vi "N147x_charge_transport.vi"() -> ()   [LabVIEW 2019]
uses:
  <vilib>/Analysis/baseanly.llb/Mean (DBL).vi
  <vilib>/Utility/file.llb/Write To Spreadsheet File (DBL).vi
  N471A.lvlib
  Users/pcmmegas02/Downloads/CAEN_PSM-InstrumentDriver-1.0.2/CAEN PSM/CAEN PSM.lvlib
  <vilib>/Analysis/NI_AALBase.lvlib
  <vilib>/gmath/NI_Gmath.lvlib
panel:
  out "seconds since 1Jan1904":timestamp
  in  "one time average":bool
  out "IMon Graph":cluster{"Y":dbl[], "Y":dbl[]}[](graph)
  out "VMon Graph":cluster{"Y":dbl[], "Y":dbl[]}[](graph)
  out "Mean-St.dev. 1":dbl[](array[numeric]) format="%#.2g"
  out "Mean-St.dev. 2":dbl[](array[numeric]) format="%#.2g"
  out "Mean-St.dev. 3":dbl[](array[numeric]) format="%#.2g"
  out "Mean-St.dev. 4":dbl[](array[numeric]) format="%#.2g"
  out "IMON RT 1":dbl[](array[numeric])
  out "IMON RT 2":dbl[](array[numeric])
  out "IMON RT 3":dbl[](array[numeric])
  out "IMON RT 4":dbl[](array[numeric])
  out "VMON RT 1":dbl[](array[numeric])
  out "VMON RT 2":dbl[](array[numeric])
  out "VMON RT 3":dbl[](array[numeric])
  out "VMON RT 4":dbl[](array[numeric])
  in  "Average length":i32=50
  out "Board Handle":T1
  in  "Save":bool
  out "Time Array":dbl[](array[numeric])=[0.09375, 0.46875, 0.84375, 1.78125, 2.15625, 2.53125, 2.921875, 3.28125, 6.09375, 6.46875, 6.859375, 7.234375, 7.609375, 7.984375, 8.359375, 8.734375, 9.109375, 9.484375, 9.859375, 10.234375, 10.625, 10.984375, 11.375, 11.75, 12.125, 12.5, 12.875, 13.25, 13.625, 14.0, 14.390625, 14.765625, 15.140625, 15.515625, 15.890625, 16.265625, 16.640625, 17.015625, 17.390625, 17.765625, 18.140625, 18.515625, 18.90625, 19.28125, 19.65625, 20.03125, 20.40625, 20.78125, 21.15625, 21.53125, 21.90625, 22.28125, 22.65625, 23.046875, 23.421875, 23.796875, 24.171875, 24.546875, 24.921875, 25.296875, 25.671875, 26.0625, 26.4375, 26.8125, 27.1875, 27.5625, 27.9375, 28.3125, 28.6875, 29.0625, 29.4375, 29.8125, 30.203125, 30.578125, 30.953125, 31.328125, 31.703125, 32.078125, 32.453125, 32.828125, 33.203125, 33.578125, 33.96875, 34.34375, 34.71875, 35.09375, 37.96875, 38.34375, 38.71875, 39.09375, 39.46875, 39.84375, 40.21875, 40.59375, 40.96875, 41.34375, 41.71875, 42.09375, 42.484375, 42.859375, 43.234375, 43.609375, 43.984375, 44.359375, 44.734375, 45.109375, 45.484375, 45.859375, 46.25, 46.625, 47.0, 47.375, 47.75, 48.125, 48.5, 48.875, 49.265625, 49.640625, 50.015625, 50.390625, 50.765625, 51.140625, 51.515625, 51.890625, 52.265625, 52.640625, 53.015625, 53.390625, 53.765625, 54.15625, 54.53125, 54.90625, 55.28125, 55.65625, 56.03125, 56.40625, 56.78125, 57.15625, 57.53125, 57.921875, 58.296875, 58.671875, 59.046875, 59.421875, 59.796875, 60.171875, 60.546875, 60.9375, 61.296875, 61.6875, 62.0625, 62.4375, 62.8125, 63.1875, 63.5625, 63.9375, 64.3125, 64.6875, 65.0625, 65.4375, 65.828125, 66.203125, 66.578125, 66.953125, 67.328125, 67.703125, 68.078125, 68.453125, 68.84375, 69.21875, 69.59375, 69.96875, 70.34375, 70.71875, 71.09375, 71.46875, 71.84375, 72.21875, 72.59375, 72.984375, 73.359375, 73.734375, 74.109375, 74.484375, 74.859375, 75.234375, 75.609375, 75.984375, 76.359375, 76.734375, 77.109375, 77.5, 77.875, 78.25, 78.625, 79.0, 79.375, 79.75, 80.125, 80.515625, 80.890625, 81.265625]
  out "IMON Array":dbl[][](array[numeric])
  out "VMON Array":dbl[][](array[numeric])
  in  "stop":bool
  in  "Module Address":u16(ring) items=["0", "1", "2", "3", "4", "5", "6", "7", "8", "9", "10", "11", "12", "13", "14", "15", "16", "17", "18", "19", "20", "21", "22", "23", "24", "25", "26", "27", "28", "29", "30", "31"]
  in  "VISA resource name in":refnum<visa-resource-name>="COM13"
  out "error out":errorcluster
  in  "N147x":T2(tab)
  in  "Read Status and Configuration":bool
  out "Name":string
  out "Number Of Channels":string
  out "Firmware Release":string
  out "Serial Number":string
  out "Channel Status Array":T3(array[cluster])
  out "PWDW":string[](array[string])
  out "Polarity":string[](array[string])
  out "MAXV":i32[](array[numeric])
  out "RDW":i32[](array[numeric])
  out "RUP":i32[](array[numeric])
  out "IMON":dbl[](array[numeric]) format="%.1f"
  out "ISET":dbl[](array[numeric]) format="%.1f"
  out "VMON":dbl[](array[numeric]) format="%.1f"
  out "VSET":dbl[](array[numeric]) format="%.1f"
  out "Number of Channel Detected":u8=4
  out "Monitoring Error":bool
  in  "IMon range":string(combo)="KILL"
  in  "Power down":string(combo)="KILL"
  in  "ALL OFF":bool
  in  "ALL ON":bool
  in  "Channels ON/OFF":bool[](array[boolean])=[TRUE, TRUE, TRUE, TRUE]
  in  "IM RANGE":bool
  in  "PDWN":bool
  in  "TRIP":bool
  in  "RDW":bool
  in  "RUP":bool
  in  "MAXV":bool
  in  "ISET[uA]":bool
  in  "VSET":bool
  in  "Channels Selection":bool[](array[boolean])=[FALSE, FALSE, FALSE, FALSE]
  in  "Upload Values":bool
  in  "Set V":dbl format="%06.1f"
  in  "Set I":dbl=2.0 format="%07.3f"
  in  "Set Max V":dbl=1000.0 format="%04.0f"
  in  "Set Ramp Up":dbl=10.0 format="%03.0f"
  in  "Set Ramp Down":dbl=50.0 format="%03.0f"
  in  "Set Trip":dbl=1000.0 format="%06.1f"
  in  "Update On/OFF":bool
  out "Error  on \nChannels \nON/OFF":bool
  out "IMon  RT Err":bool
  out "VMon  RT Err":bool
  in  "stop HV scan":bool
  in  "Waiting [s]":u32=7
  in  "Step [V]":dbl[](array[numeric])=[50.0, 50.0] format="%06.1f"
  in  "Vstop":dbl[](array[numeric])=[1600.0, 1600.0, 10.0, 10.0] format="%06.1f"
  in  "Channels Selection 2":bool[](array[boolean])=[FALSE, FALSE, FALSE, FALSE]
  in  "Start HV scan":bool
  in  "Vstart":dbl[](array[numeric])=[0.0, 0.0, 10.0, 10.0] format="%06.1f"
  in  "pts/step":i32=5
  out "logged pts/step":i32
  out "Scatter Plot":cluster{dbl[], dbl[]}[](graph)=[{[199.2, 172.7, 149.1, 124.2, 99.2, 74.2, 49.19999999999999, 24.30000000000001, -0.5999999999999943, -25.5, -50.5, -75.39999999999998, -100.39999999999998, -125.5, -150.3, -175.2, -200.2, -225.2, -250.10000000000002, -275.1, -300.2, -325.0, -350.0, -375.0, -399.9, -424.70000000000005, -449.70000000000005, -474.6, -499.70000000000005, -524.8000000000001, -549.8000000000001, -574.6, -599.4, -599.6, -599.6, -599.6, -599.6, -599.6, -599.6], [0.0, 0.0, 0.0, 0.0, 0.0, 0.0, 0.0, 0.05, 0.05, 0.05, 0.05, 0.15, 0.1, 0.15, 0.15, 0.15, 0.15, 0.2, 0.2, 0.25, 0.25, 0.3, 0.35, 0.4, 0.4, 0.4, 0.45, 0.5, 0.45, 0.5, 0.55, 0.6, 0.6, 0.6, 0.65, 0.6, 0.6, 0.6, 0.6]}, {[199.2, 172.7, 149.1, 124.2, 99.2, 74.2, 49.19999999999999, 24.30000000000001, -0.5999999999999943, -25.5, -50.5, -75.39999999999998, -100.39999999999998, -125.5, -150.3, -175.2, -200.2, -225.2, -250.10000000000002, -275.1, -300.2, -325.0, -350.0, -375.0, -399.9, -424.70000000000005, -449.70000000000005, -474.6, -499.70000000000005, -524.8000000000001, -549.8000000000001, -574.6, -599.4, -599.6, -599.6, -599.6, -599.6, -599.6, -599.6], [0.1, 0.25, 0.15, 0.15, 0.15, 0.2, 0.2, 0.25, 0.25, 0.25, 0.25, 0.3, 0.35, 0.4, 0.4, 0.45, 0.5, 0.5, 0.6, 0.65, 0.75, 0.9, 1.0, 1.15, 1.3, 1.5, 1.8, 2.1, 2.4499999999999997, 2.9499999999999997, 3.4499999999999997, 4.2, 5.05, 5.05, 5.05, 5.05, 5.1000000000000005, 5.15, 5.1000000000000005]}, {[199.2, 172.7, 149.1, 124.2, 99.2, 74.2, 49.19999999999999, 24.30000000000001, -0.5999999999999943, -25.5, -50.5, -75.39999999999998, -100.39999999999998, -125.5, -150.3, -175.2, -200.2, -225.2, -250.10000000000002, -275.1, -300.2, -325.0, -350.0, -375.0, -399.9, -424.70000000000005, -449.70000000000005, -474.6, -499.70000000000005, -524.8000000000001, -549.8000000000001, -574.6, -599.4, -599.6, -599.6, -599.6, -599.6, -599.6, -599.6], [0.0, 0.6, 0.05, 0.05, 0.05, 0.05, 0.05, 0.05, 0.05, 0.1, 0.1, 0.1, 0.15, 0.1, 0.15, 0.15, 0.15, 0.15, 0.15, 0.2, 0.2, 0.25, 0.25, 0.3, 0.35, 0.45, 0.5, 0.6, 0.7, 0.8, 1.0, 1.2, 1.55, 1.5, 1.5, 1.45, 1.5, 1.45, 1.45]}, {[199.2, 172.7, 149.1, 124.2, 99.2, 74.2, 49.19999999999999, 24.30000000000001, -0.5999999999999943, -25.5, -50.5, -75.39999999999998, -100.39999999999998, -125.5, -150.3, -175.2, -200.2, -225.2, -250.10000000000002, -275.1, -300.2, -325.0, -350.0, -375.0, -399.9, -424.70000000000005, -449.70000000000005, -474.6, -499.70000000000005, -524.8000000000001, -549.8000000000001, -574.6, -599.4, -599.6, -599.6, -599.6, -599.6, -599.6, -599.6], [0.0, 0.05, 0.1, 0.1, 0.25, 0.25, 0.25, 0.25, 0.25, 0.35, 0.35, 0.45, 0.45, 0.45, 0.5, 0.55, 0.65, 0.7, 0.8, 0.9, 0.95, 1.05, 1.2, 1.35, 1.45, 1.7, 1.9, 2.15, 2.4499999999999997, 2.8, 3.2, 3.75, 4.35, 4.3, 4.3, 4.25, 4.3, 4.3, 4.3]}]
  in  "Average values":bool
  # "Channel 1               Channel 2              Channel 3               Channel 4"
  # "VMON RT [V]"
  # "IMON RT (nA)"
  # "Mean value (nA)"
  # "St. dev."
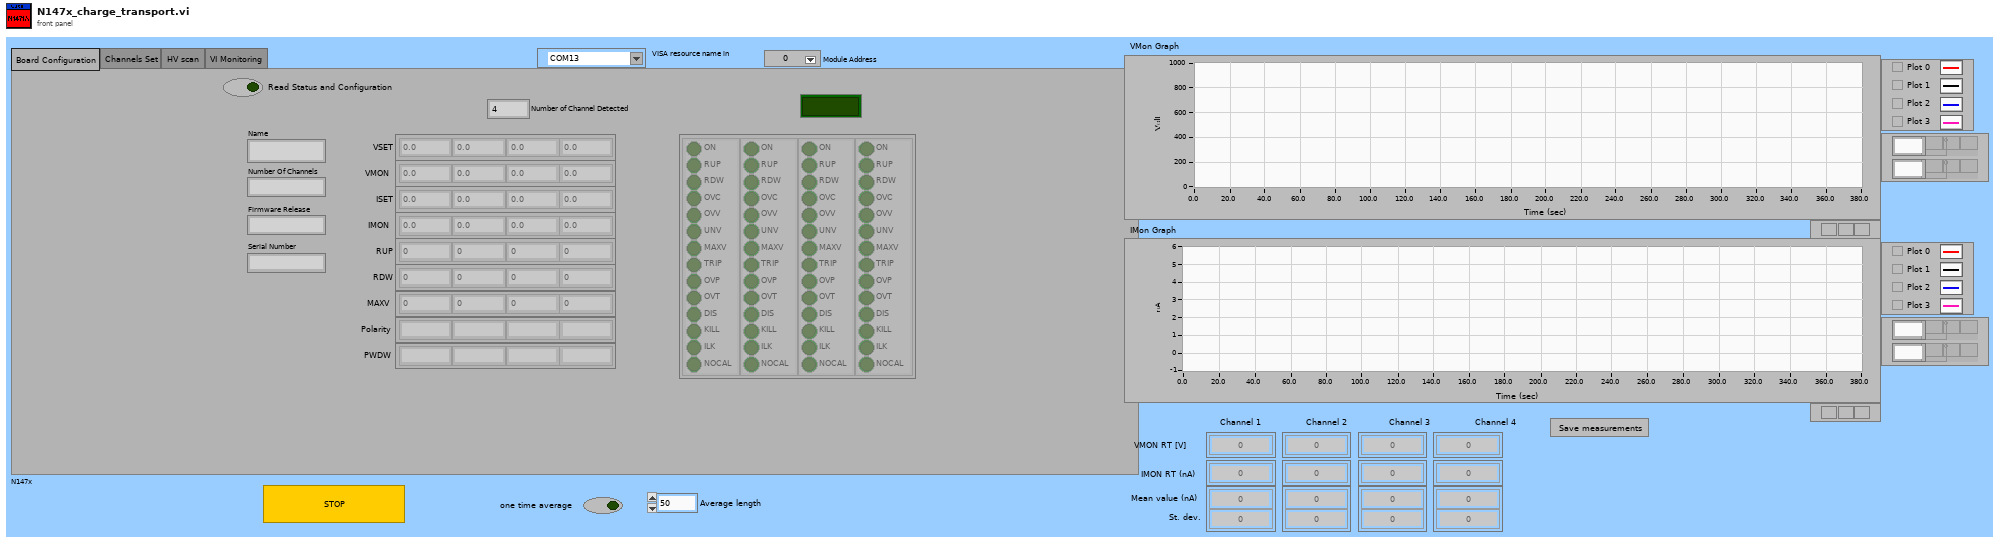
[diagram p1: front panel]
types:
  T1 = cluster{"VISA resource name in":refnum<visa-resource-name>, "Module Address":u16, "Number of Channel Detected":u8}
  T2 = enum32{"Board Configuration", "Channels Set", "HV scan", "VI Monitoring"}
  T3 = cluster{"ON":bool, "RUP":bool, "RDW":bool, "OVC":bool, "OVV":bool, "UNV":bool, "MAXV":bool, "TRIP":bool, "OVP":bool, "OVT":bool, "DIS":bool, "KILL":bool, "ILK":bool, "NOCAL":bool}[]
  T4 = cluster{"Name":string, "Num. Channels":string, "Firmware Release":string, "Serial Num.":string}
  T5 = typedef "CAEN PSM.lvlib/BoardHandle.ctl" = cluster{"VISA resource name":refnum<visa-resource-name>, "Board address":u8, "NChannels":u8}
  T6 = cluster{"ON":bool, "RUP":bool, "RDW":bool, "OVC":bool, "OVV":bool, "UNV":bool, "MAXV":bool, "TRIP":bool, "OVP":bool, "OVT":bool, "DIS":bool, "KILL":bool, "ILK":bool, "NOCAL":bool}
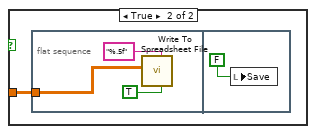
[diagram p3: hidden frame]
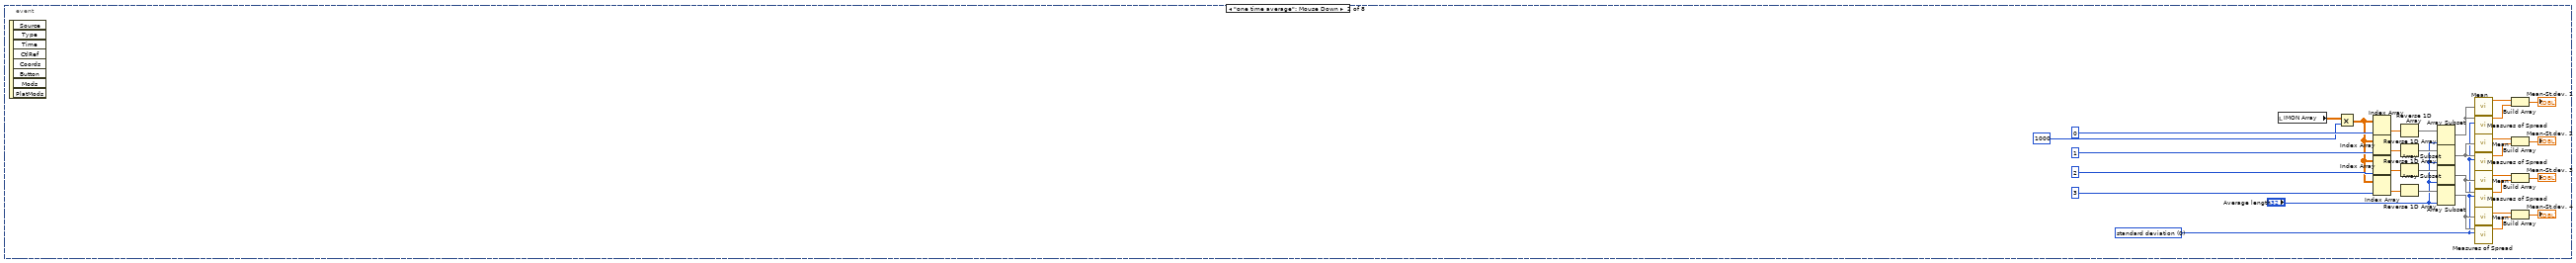
[diagram p4: hidden frame]
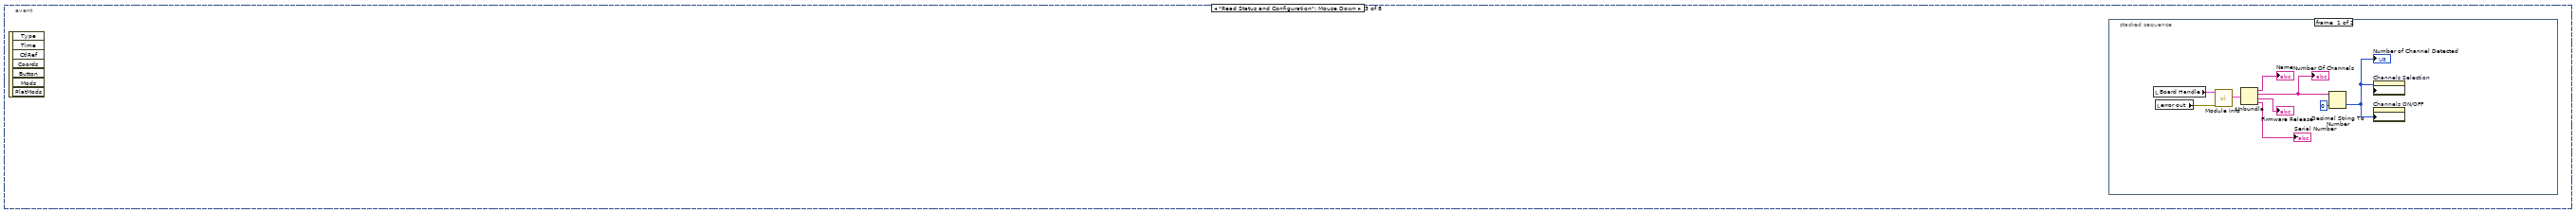
[diagram p5: hidden frame]
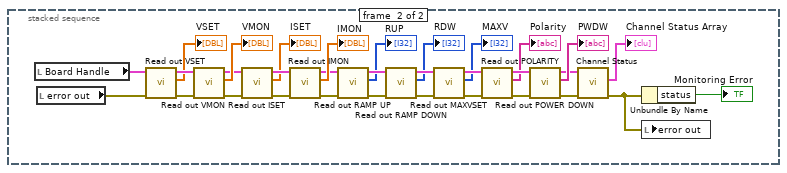
[diagram p6: hidden frame]
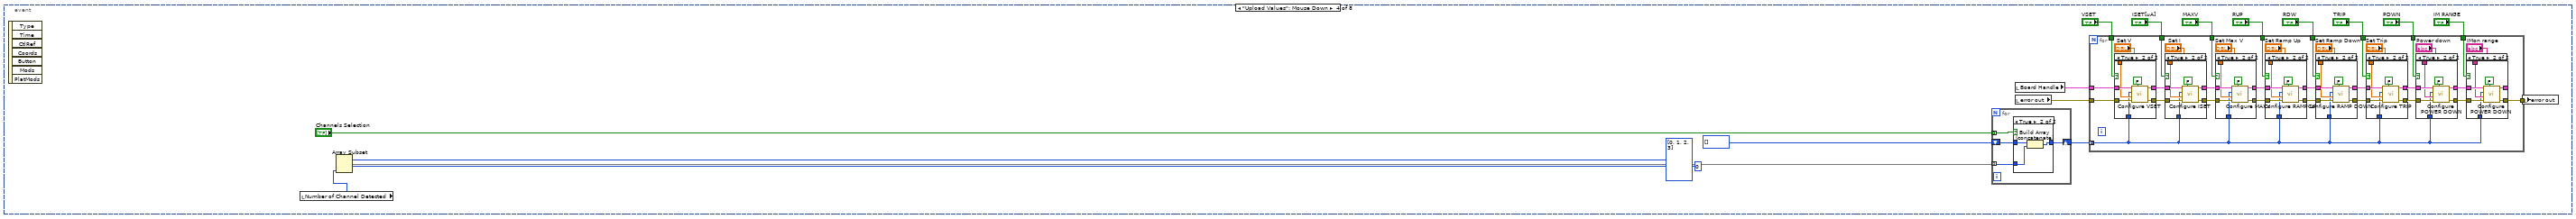
[diagram p7: hidden frame]
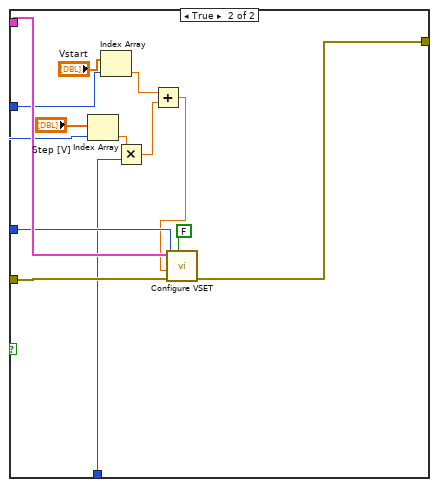
[diagram p18: hidden frame]
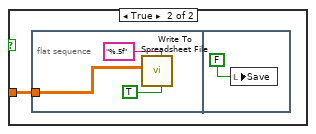
[diagram p19: hidden frame]
diagram:
  n1 = call "Initialize.vi"("VISA resource name"="VISA resource name in") -> ("error out"=w13:errorcluster, "VISA resource name out"=w9:refnum<visa-resource-name>)  [unwired: 9 in]
  n2 = local read "Number of Channel Detected"() -> (w6:u8)
  n3 = local read "VISA resource name in"() -> (w7:refnum<visa-resource-name>)
  n4 = local read "Module Address"() -> (w5:u16)
  n5 = call "OpenBoard.vi"("error in (no error)"=w13, "Board Address"=w5, "VISA resource name"=w9) -> ("error out"=w10:errorcluster)  [unwired: 7 in, 1 out]
  n6 = flat-sequence {
    tunnel: w10 -> [w17]
    tunnel: [w16] -> w11
    tunnel: [w22] -> w12
    tunnel: w11 -> [w22]
    tunnel: [w20] -> w1
    frame #0 {
      n7 = call "Display Message to User"("error in (no error)"=w17) -> ("error out"=w16:errorcluster)  [unwired: 9 in, 1 out]
    }
    frame #1 {
      w19 = dbl[][] [] ("VMON Array")
      n8 = local write "VMON Array"(w19) -> ()
      n9 = local write "IMON Array"(w19) -> ()
      n10 = local write "Time Array"(dbl[] [] ("Time Array")) -> ()
      n11 = local write "N147x"(enum32{"Board Configuration", "Channels Set"}."Board Configuration" ("N1471A 2")) -> ()
      n12 = Get Date/Time In Seconds() -> (seconds since 1Jan1904=w20:timestamp)
    }
  }
  n13 = Bundle("VISA resource name in"=w7, "Module Address"=w5, "Number of Channel Detected"=w6) -> (w8:T1)  [unwired: 1 in]
  "Board Handle" <- w8
  n14 = local write "Board Handle"(w8) -> ()
  n15 = while {
    shift-right: [w23] -> w4
    shift-left: w12 -> [w28]
    tunnel: [FALSE ("stop")] -> w15
    stop <- w26 stop-if-true
    n16 = flat-sequence {
      tunnel: w28 -> [w30]
      tunnel: [w30] -> w29
      frame #0 {
        n17 = local write "error out"(w30) -> ()
      }
    }
    n18 = case shown="No Error" w29 {
      selector: w29 -> [_ w821]
      tunnel: [w31 w821] -> w23
      frame No Error {
        n19 = event shown="[4] \"Start HV scan\": Mouse Down" {
          selector: _ -> [_ _ _ _ _ _ _ _]
          dyn-events: _ -> [_ _ _ _ _ _ _ _]
          timeout: u32 1 ("Time") -> [_ _ _ _ _ _ _ _]
          tunnel: [w100 _ _ _ _ _ _ _] -> w31
          event Timeout {
            w91 = cluster{dbl[], dbl[]}[] []
            w99 = FALSE ("Open/Close [T]")
            n20 = event-data() -> ()  [unwired: 1 in, 2 out]
            n21 = local read "Number of Channel Detected"() -> (w88:u8)
            n22 = local read "seconds since 1Jan1904"() -> (w33:timestamp)
            n23 = Get Date/Time In Seconds() -> (seconds since 1Jan1904=w95:timestamp)
            n24 = local read "VISA resource name in"() -> (w103:refnum<visa-resource-name>)
            n25 = local read "Module Address"() -> (w98:u16)
            n26 = local read "VMON Array"() -> (w87:dbl[][])
            n27 = local read "IMON Array"() -> (w92:dbl[][])
            n28 = Subtract(x=w95, y=w33) -> (x-y=w89:dbl)
            n29 = local read "Time Array"() -> (w90:dbl[])
            n30 = Wait Until Next ms Multiple(millisecond multiple=u32 1000 ("milliseconds to wait")) -> ()  [unwired: 1 out]
            n31 = Build Array (concatenate)(w90, w89) -> (w75:dbl[])
            n32 = local write "Time Array"(w75) -> ()
            n33 = local read "error out"() -> (w63:errorcluster)
            n34 = call "N1471A-MonitorVMON.vi"("VISA resource name in"=w103, "Module Address"=w98, "Channel"=w88, "error in (no error)"=w63, "Open/Close [T]"=w99) -> ("VISA resource name out"=w102:refnum<visa-resource-name>, "Error"=→"VMon  RT Err":bool, "Values"=w94:string[], "error out"=w101:errorcluster)  [unwired: 9 in, 2 out]
            n35 = call "N1471A-MonitorIMON.vi"("VISA resource name in"=w102, "Module Address"=w98, "Channel"=w88, "error in (no error)"=w101, "Open/Close [T]"=w99) -> ("Error"=→"IMon  RT Err":bool, "Values"=w93:string[], "error out"=w100:errorcluster)  [unwired: 9 in, 3 out]
            n36 = for {
              N: w88 -> [_]
              tunnel: w94 -> [w130] mode=indexing
              tunnel: w93 -> [w127] mode=indexing
              tunnel: [w129] -> w34 mode=indexing
              tunnel: [w128] -> w53 mode=indexing
              tunnel: w92 -> [w122]
              tunnel: w87 -> [w124]
              i -> [w121]
              n37 = Index Array(array=w124, index (col)=w121) -> (element=w123:dbl[])  [unwired: 1 in]
              n38 = Index Array(array=w122, index (col)=w121) -> (element=w120:dbl[])  [unwired: 1 in]
              n39 = Fract/Exp String To Number(string=w130) -> (number=w126:dbl)  [unwired: 3 in, 1 out]
              n40 = Fract/Exp String To Number(string=w127) -> (number=w125:dbl)  [unwired: 3 in, 1 out]
              n41 = Build Array (concatenate)(w123, w126) -> (w129:dbl[])
              n42 = Build Array (concatenate)(w120, w125) -> (w128:dbl[])
            }
            n43 = Multiply(x=w53, y=1000) -> (x*y=w48:dbl[][])
            n44 = Index Array(array=w34, index (row) #1=0 ("index (row)"), index (row) #2=1 ("index (row)"), index (row) #3=2 ("index (row)"), index (row) #4=3 ("index (row)")) -> (element #1=w74:dbl[], element #2=w72:dbl[], element #3=w70:dbl[], element #4=w68:dbl[])  [unwired: 4 in]
            n45 = Index Array(array=w53, index (row) #1=0 ("index (row)"), index (row) #2=1 ("index (row)"), index (row) #3=2 ("index (row)"), index (row) #4=3 ("index (row)")) -> (element #1=w73:dbl[], element #2=w71:dbl[], element #3=w69:dbl[], element #4=w67:dbl[])  [unwired: 4 in]
            n46 = Transpose 2D Array(2D array=w34) -> (transposed array=w86:dbl[][])
            n47 = Transpose 2D Array(2D array=w53) -> (transposed array=w62:dbl[][])
            n48 = Index Array(array=w48, index (row) #1=0 ("index (row)"), index (row) #2=1 ("index (row)"), index (row) #3=2 ("index (row)"), index (row) #4=3 ("index (row)")) -> (element #1=w57:dbl[], element #2=w56:dbl[], element #3=w55:dbl[], element #4=w54:dbl[])  [unwired: 4 in]
            n49 = Build Array(w75, w74, w73, w72, w71, w70, w69, w68, w67) -> (w66:dbl[][])
            n50 = local write "VMON Array"(w86) -> ()
            n51 = local write "IMON Array"(w62) -> ()
            n52 = Reverse 1D Array(array=w57) -> (reversed array=→"IMON RT 1":dbl[])
            n53 = Reverse 1D Array(array=w56) -> (reversed array=→"IMON RT 2":dbl[])
            n54 = Reverse 1D Array(array=w55) -> (reversed array=→"IMON RT 3":dbl[])
            n55 = Reverse 1D Array(array=w54) -> (reversed array=→"IMON RT 4":dbl[])
            n56 = case shown="False" "Save" {
              tunnel: w66 -> [_ w104]
              frame False {
              }
              frame True {
                n57 = flat-sequence {
                  tunnel: w104 -> [w106]
                  frame #0 {
                    n58 = call-poly <vilib>:"Write To Spreadsheet File.vi"("transpose? (no:F)"=TRUE, "format (%.3f)"="%.5f", "2D data"=w106) -> ()  [unwired: 5 in, 1 out]
                  }
                  frame #1 {
                    n59 = local write "Save"(FALSE ("Save")) -> ()
                  }
                }
              }
            }
            n60 = for {
              tunnel: w34 -> [w115] mode=indexing
              shift-right: [w119] -> w64
              shift-left: w91 -> [w118]
              shift-right: [w117] -> w85
              shift-left: w91 -> [w116]
              tunnel: w53 -> [w114] mode=indexing
              tunnel: w75 -> [w113]
              n61 = Multiply(x=w114, y=1000) -> (x*y=w110:dbl[])
              n62 = Bundle(w113, w115) -> (w112:cluster{dbl[], dbl[]})  [unwired: 1 in]
              n63 = Bundle(w113, w110) -> (w111:cluster{dbl[], dbl[]})  [unwired: 1 in]
              n64 = Build Array (concatenate)(w118, w112) -> (w119:cluster{dbl[], dbl[]}[])
              n65 = Build Array (concatenate)(w116, w111) -> (w117:cluster{dbl[], dbl[]}[])
            }
            "IMon Graph" <- w85
            "VMon Graph" <- w64
            n66 = Index Array(array=w34, index (row) #1=0 ("index (row)"), index (row) #2=1 ("index (row)"), index (row) #3=2 ("index (row)"), index (row) #4=3 ("index (row)")) -> (element #1=w42:dbl[], element #2=w41:dbl[], element #3=w40:dbl[], element #4=w39:dbl[])  [unwired: 4 in]
            n67 = Reverse 1D Array(array=w42) -> (reversed array=→"VMON RT 1":dbl[])
            n68 = Reverse 1D Array(array=w41) -> (reversed array=→"VMON RT 2":dbl[])
            n69 = Reverse 1D Array(array=w40) -> (reversed array=→"VMON RT 3":dbl[])
            n70 = Reverse 1D Array(array=w39) -> (reversed array=→"VMON RT 4":dbl[])
          }
          event "one time average": Mouse Down {
            w133 = 0 items=["standard deviation", "range", "mean absolute deviation", "interquartile range"] ("type")
            n71 = event-data() -> ()  [unwired: 1 in, 8 out]
            n72 = local read "IMON Array"() -> (w132:dbl[][])
            n73 = Multiply(x=w132, y=1000) -> (x*y=w134:dbl[][])
            n74 = Index Array(array=w134, index (col)=0 ("disabled index (col)")) -> (element=w159:dbl[])  [unwired: 1 in]
            n75 = Index Array(array=w134, index (col)=1 ("disabled index (col)")) -> (element=w158:dbl[])  [unwired: 1 in]
            n76 = Index Array(array=w134, index (col)=2 ("disabled index (col)")) -> (element=w157:dbl[])  [unwired: 1 in]
            n77 = Index Array(array=w134, index (col)=3 ("disabled index (col)")) -> (element=w156:dbl[])  [unwired: 1 in]
            n78 = Reverse 1D Array(array=w159) -> (reversed array=w154:dbl[])
            n79 = Reverse 1D Array(array=w158) -> (reversed array=w153:dbl[])
            n80 = Reverse 1D Array(array=w157) -> (reversed array=w152:dbl[])
            n81 = Reverse 1D Array(array=w156) -> (reversed array=w151:dbl[])
            n82 = Array Subset(array=w154, length="Average length") -> (w143:dbl[])  [unwired: 1 in]
            n83 = Array Subset(array=w153, length="Average length") -> (w146:dbl[])  [unwired: 1 in]
            n84 = Array Subset(array=w152, length="Average length") -> (w145:dbl[])  [unwired: 1 in]
            n85 = Array Subset(array=w151, length="Average length") -> (w144:dbl[])  [unwired: 1 in]
            n86 = call-poly <vilib>:"Mean.vi"("X"=w143) -> ("mean"=w142:dbl)  [unwired: 1 out]
            n87 = call <vilib>:"Measures of Spread.vi"("type"=w133, "x array"=w143) -> ("spread value"=w141:dbl)  [unwired: 8 in, 1 out]
            n88 = call-poly <vilib>:"Mean.vi"("X"=w146) -> ("mean"=w140:dbl)  [unwired: 1 out]
            n89 = call <vilib>:"Measures of Spread.vi"("type"=w133, "x array"=w146) -> ("spread value"=w139:dbl)  [unwired: 8 in, 1 out]
            n90 = call-poly <vilib>:"Mean.vi"("X"=w145) -> ("mean"=w138:dbl)  [unwired: 1 out]
            n91 = call <vilib>:"Measures of Spread.vi"("type"=w133, "x array"=w145) -> ("spread value"=w137:dbl)  [unwired: 8 in, 1 out]
            n92 = call-poly <vilib>:"Mean.vi"("X"=w144) -> ("mean"=w136:dbl)  [unwired: 1 out]
            n93 = call <vilib>:"Measures of Spread.vi"("type"=w133, "x array"=w144) -> ("spread value"=w135:dbl)  [unwired: 8 in, 1 out]
            n94 = Build Array(w142, w141) -> (→"Mean-St.dev. 1":dbl[])
            n95 = Build Array(w140, w139) -> (→"Mean-St.dev. 2":dbl[])
            n96 = Build Array(w138, w137) -> (→"Mean-St.dev. 3":dbl[])
            n97 = Build Array(w136, w135) -> (→"Mean-St.dev. 4":dbl[])
          }
          event "Read Status and Configuration": Mouse Down {
            n98 = event-data() -> ()  [unwired: 1 in, 7 out]
            n99 = stacked-sequence {
              frame #0 {
                n100 = local read "Board Handle"() -> (w164:T1)
                n101 = local read "error out"() -> (w165:errorcluster)
                n102 = call "Module Info.vi"("error in (no error)"=w165, "BoardHandle"=w164) -> ("Module Info"=w170:T4)  [unwired: 7 in, 2 out]
                n103 = Unbundle(w170) -> ("Name"=→"Name":string, "Num. Channels"=w168:string, "Firmware Release"=→"Firmware Release":string, "Serial Num."=→"Serial Number":string)
                "Number Of Channels" <- w168
                n104 = Decimal String To Number(string=w168, default (0L)=u8 0 ("default (0 I32)")) -> (number=w171:u8)  [unwired: 1 in, 1 out]
                "Number of Channel Detected" <- w171
                n105 = property on="Channels Selection" class="Arr (strict)"("Number of Columns"=w171) -> ()  [unwired: 2 in, 2 out]
                n106 = property on="Channels ON/OFF" class="Arr (strict)"("Number of Columns"=w171) -> ()  [unwired: 2 in, 2 out]
              }
              frame #1 {
                n107 = local read "Board Handle"() -> (w173:T1)
                n108 = local read "error out"() -> (w194:errorcluster)
                n109 = call "Read out VSET.vi"("error in (no error)"=w194, "BoardHandle"=w173) -> ("error out"=w203:errorcluster, "Vset values (V)"=→"VSET":dbl[], "BoardHandle out"=w204:T5)  [unwired: 6 in, 1 out]
                n110 = call "Read out VMON.vi"("error in (no error)"=w203, "BoardHandle"=w204) -> ("error out"=w199:errorcluster, "VMon values (V)"=→"VMON":dbl[], "BoardHandle out"=w200:T5)  [unwired: 7 in]
                n111 = call "Read out ISET.vi"("error in (no error)"=w199, "BoardHandle"=w200) -> ("error out"=w198:errorcluster, "ISet values (uA)"=→"ISET":dbl[], "BoardHandle out"=w197:T5)  [unwired: 6 in, 1 out]
                n112 = call "Read out IMON.vi"("error in (no error)"=w198, "BoardHandle"=w197) -> ("error out"=w193:errorcluster, "IMon values (uA)"=→"IMON":dbl[], "BoardHandle out"=w192:T5)  [unwired: 6 in, 1 out]
                n113 = call "Read out RAMP UP.vi"("error in (no error)"=w193, "BoardHandle"=w192) -> ("error out"=w191:errorcluster, "Ramp up values  (V/s)"=→"RUP":i32[], "BoardHandle out"=w190:T5)  [unwired: 6 in, 1 out]
                n114 = call "Read out RAMP DOWN.vi"("error in (no error)"=w191, "BoardHandle"=w190) -> ("error out"=w189:errorcluster, "Ramp down values  (V/s)"=→"RDW":i32[], "BoardHandle out"=w188:T5)  [unwired: 6 in, 1 out]
                n115 = call "Read out MAXVSET.vi"("error in (no error)"=w189, "BoardHandle"=w188) -> ("error out"=w187:errorcluster, "Voltage max values (V)"=→"MAXV":i32[], "BoardHandle out"=w186:T5)  [unwired: 6 in, 1 out]
                n116 = call "Read out POLARITY.vi"("error in (no error)"=w187, "BoardHandle"=w186) -> ("error out"=w185:errorcluster, "Polarity values"=→"Polarity":string[], "BoardHandle out"=w184:T5)  [unwired: 7 in]
                n117 = call "Read out POWER DOWN.vi"("error in (no error)"=w185, "BoardHandle"=w184) -> ("error out"=w176:errorcluster, "Power down values"=→"PWDW":string[], "BoardHandle out"=w177:T5)  [unwired: 7 in]
                n118 = call "Channel Status.vi"("error in (no error)"=w176, "BoardHandle"=w177) -> ("error out"=w175:errorcluster, "Channel Status Array"=→"Channel Status Array":T3)  [unwired: 7 in, 1 out]
                n119 = Unbundle By Name(w175) -> ("status"=→"Monitoring Error":bool)
                n120 = local write "error out"(w175) -> ()
              }
            }
          }
          event "Upload Values": Mouse Down {
            n121 = event-data() -> ()  [unwired: 1 in, 7 out]
            n122 = local read "Number of Channel Detected"() -> (w218:u8)
            n123 = Array Subset(array=u8[] [0, 1, 2, 3], index=0, length=w218) -> (w220:u8[])
            n124 = for {
              shift-right: [w331] -> w215
              shift-left: u8[] [] -> [w332]
              tunnel: w220 -> [w330] mode=indexing
              tunnel: "Channels Selection" -> [w329] mode=indexing
              n125 = case shown="True" w329 {
                tunnel: w332 -> [w333 w336]
                tunnel: [w333 w335] -> w331
                tunnel: w330 -> [_ w334]
                frame False {
                }
                frame True {
                  n126 = Build Array (concatenate)(w336, w334) -> (w335:u8[])
                }
              }
            }
            n127 = local read "Board Handle"() -> (w217:T1)
            n128 = local read "error out"() -> (w216:errorcluster)
            n129 = for {
              tunnel: w217 -> [w256]
              tunnel: w216 -> [w255]
              tunnel: w215 -> [w232] mode=indexing
              tunnel: [w231] -> w213
              tunnel: "VSET" -> [w230]
              tunnel: "ISET[uA]" -> [w229]
              tunnel: "MAXV" -> [w228]
              tunnel: "RUP" -> [w227]
              tunnel: "RDW" -> [w226]
              tunnel: "TRIP" -> [w225]
              tunnel: "PDWN" -> [w224]
              tunnel: "IM RANGE" -> [w223]
              n130 = case shown="True" w230 {
                tunnel: w255 -> [w321 w323]
                tunnel: w256 -> [w320 w327]
                tunnel: [w320 w326] -> w254
                tunnel: [w321 w325] -> w253
                tunnel: "Set V" -> [_ w324]
                tunnel: w232 -> [_ w322]
                frame False {
                }
                frame True {
                  n131 = call "Configure VSET.vi"("All Channels (F)"=FALSE, "error in (no error)"=w323, "Voltage Level (0.0 V)"=w324, "Channel (0)"=w322, "BoardHandle"=w327) -> ("error out"=w325:errorcluster, "BoardHandle out"=w326:T5)  [unwired: 5 in]
                }
              }
              n132 = case shown="True" w229 {
                tunnel: w253 -> [w312 w314]
                tunnel: w254 -> [w311 w318]
                tunnel: [w311 w317] -> w250
                tunnel: [w312 w316] -> w249
                tunnel: "Set I" -> [_ w315]
                tunnel: w232 -> [_ w313]
                frame False {
                }
                frame True {
                  n133 = call "Configure ISET.vi"("All Channels (F)"=FALSE, "error in (no error)"=w314, "Current Limit (0.00 uA)"=w315, "Channel (0)"=w313, "BoardHandle"=w318) -> ("error out"=w316:errorcluster, "BoardHandle out"=w317:T5)  [unwired: 5 in]
                }
              }
              n134 = case shown="True" w228 {
                tunnel: w249 -> [w303 w305]
                tunnel: w250 -> [w302 w309]
                tunnel: [w302 w308] -> w248
                tunnel: [w303 w307] -> w247
                tunnel: "Set Max V" -> [_ w306]
                tunnel: w232 -> [_ w304]
                frame False {
                }
                frame True {
                  n135 = call "Configure MAXV.vi"("All Channels (F)"=FALSE, "error in (no error)"=w305, "Voltage Max (0.0 V)"=w306, "Channel (0)"=w304, "BoardHandle"=w309) -> ("error out"=w307:errorcluster, "BoardHandle out"=w308:T5)  [unwired: 5 in]
                }
              }
              n136 = case shown="True" w227 {
                tunnel: w247 -> [w294 w296]
                tunnel: w248 -> [w293 w300]
                tunnel: [w293 w299] -> w246
                tunnel: [w294 w298] -> w245
                tunnel: "Set Ramp Up" -> [_ w297]
                tunnel: w232 -> [_ w295]
                frame False {
                }
                frame True {
                  n137 = call "Configure RAMP UP.vi"("All Channels (F)"=FALSE, "error in (no error)"=w296, "Voltage ramp up (0 V/s)"=w297, "Channel (0)"=w295, "BoardHandle"=w300) -> ("error out"=w298:errorcluster, "BoardHandle out"=w299:T5)  [unwired: 5 in]
                }
              }
              n138 = case shown="True" w226 {
                tunnel: w245 -> [w285 w287]
                tunnel: w246 -> [w284 w291]
                tunnel: [w284 w290] -> w244
                tunnel: [w285 w289] -> w243
                tunnel: "Set Ramp Down" -> [_ w288]
                tunnel: w232 -> [_ w286]
                frame False {
                }
                frame True {
                  n139 = call "Configure RAMP DOWN.vi"("All Channels (F)"=FALSE, "error in (no error)"=w287, "Voltage ramp down (0 V/s)"=w288, "Channel (0)"=w286, "BoardHandle"=w291) -> ("error out"=w289:errorcluster, "BoardHandle out"=w290:T5)  [unwired: 5 in]
                }
              }
              n140 = case shown="True" w225 {
                tunnel: w243 -> [w276 w278]
                tunnel: w244 -> [w275 w282]
                tunnel: [w275 w281] -> w242
                tunnel: [w276 w280] -> w241
                tunnel: "Set Trip" -> [_ w279]
                tunnel: w232 -> [_ w277]
                frame False {
                }
                frame True {
                  n141 = call "Configure TRIP.vi"("All Channels (F)"=FALSE, "error in (no error)"=w278, "Trip (0.00 s)"=w279, "Channel (0)"=w277, "BoardHandle"=w282) -> ("error out"=w280:errorcluster, "BoardHandle out"=w281:T5)  [unwired: 5 in]
                }
              }
              n142 = case shown="True" w224 {
                tunnel: w241 -> [w267 w270]
                tunnel: w242 -> [w266 w273]
                tunnel: [w266 w272] -> w234
                tunnel: [w267 w271] -> w233
                tunnel: "Power down" -> [_ w269]
                tunnel: w232 -> [_ w268]
                frame False {
                }
                frame True {
                  n143 = call "Configure POWER DOWN.vi"("All Channels (F)"=FALSE, "error in (no error)"=w270, "Power down (KILL)"=w269, "Channel (0)"=w268, "BoardHandle"=w273) -> ("error out"=w271:errorcluster, "BoardHandle out"=w272:T5)  [unwired: 5 in]
                }
              }
              n144 = case shown="True" w223 {
                tunnel: w233 -> [w258 w261]
                tunnel: w234 -> [w257 w264]
                tunnel: [w257 w263] -> _
                tunnel: [w258 w262] -> w231
                tunnel: "IMon range" -> [_ w260]
                tunnel: w232 -> [_ w259]
                frame False {
                }
                frame True {
                  n145 = call "Configure POWER DOWN.vi"("All Channels (F)"=FALSE, "error in (no error)"=w261, "Power down (KILL)"=w260, "Channel (0)"=w259, "BoardHandle"=w264) -> ("error out"=w262:errorcluster, "BoardHandle out"=w263:T5)  [unwired: 5 in]
                }
              }
            }
            n146 = local write "error out"(w213) -> ()
          }
          event "Start HV scan": Mouse Down {
            w347 = dbl[][] []  # IMON Array scan
            w348 = dbl[][] []  # VMON Array scan
            n147 = event-data() -> ()  [unwired: 1 in, 8 out]
            n148 = local read "Number of Channel Detected"() -> (w337:u8)
            n149 = local read "Module Address"() -> (w344:u16)
            n150 = local read "VISA resource name in"() -> (w346:refnum<visa-resource-name>)
            n151 = local read "error out"() -> (w345:errorcluster)
            n152 = local read "Number of Channel Detected"() -> (w353:u8)
            n153 = Array Subset(array=u8[] [0, 1, 2, 3], index=0, length=w353) -> (w355:u8[])
            n154 = call "N1471A-MonitorIMON.vi"("VISA resource name in"=w346, "Module Address"=w344, "Channel"=w337, "error in (no error)"=w345, "Open/Close [T]"=FALSE) -> ("Values"=w342:string[])  [unwired: 9 in, 5 out]
            n155 = for {
              shift-right: [w635] -> w351
              shift-left: u8[] [] -> [w636]
              tunnel: w355 -> [w634] mode=indexing
              tunnel: "Channels Selection 2" -> [w633] mode=indexing
              n156 = case shown="True" w633 {
                tunnel: w636 -> [w637 w640]
                tunnel: [w637 w639] -> w635
                tunnel: w634 -> [_ w638]
                frame False {
                }
                frame True {
                  n157 = Build Array (concatenate)(w640, w638) -> (w639:u8[])
                }
              }
            }
            n158 = call "N1471A-MonitorVMON.vi"("VISA resource name in"=w346, "Module Address"=w344, "Channel"=w337, "error in (no error)"=w345, "Open/Close [T]"=FALSE) -> ("Values"=w343:string[])  [unwired: 9 in, 5 out]
            n159 = for {
              tunnel: w343 -> [w364] mode=indexing
              tunnel: w342 -> [w363] mode=indexing
              tunnel: [w361] -> w341 mode=indexing
              tunnel: [w358] -> w340 mode=indexing
              i -> [w359]
              n160 = Fract/Exp String To Number(string=w364) -> (number=w362:dbl)  [unwired: 3 in, 1 out]
              n161 = Fract/Exp String To Number(string=w363) -> (number=w360:dbl)  [unwired: 3 in, 1 out]
              n162 = Initialize Array(w362, w359) -> (w361:dbl[])
              n163 = Initialize Array(w360, w359) -> (w358:dbl[])
            }
            n164 = local read "error out"() -> (w349:errorcluster)
            n165 = local read "Board Handle"() -> (w352:T1)
            n166 = while {
              tunnel: w352 -> [w398]
              tunnel: w351 -> [w397]
              tunnel: w349 -> [w395]
              shift-right: [w367] -> _
              shift-left: w348 -> [w388]
              shift-right: [w368] -> _
              shift-left: w347 -> [w384]
              shift-right: [w366] -> _
              shift-left: w341 -> [w380]
              shift-right: [w365] -> _
              shift-left: w340 -> [w377]
              i -> [w399]
              stop <- "stop HV scan" stop-if-true
              n167 = flat-sequence {
                tunnel: w397 -> [w404]
                tunnel: w398 -> [w405]
                tunnel: w399 -> [w406]
                tunnel: w395 -> [w407]
                tunnel: [w407] -> w394
                tunnel: [w406] -> w393
                tunnel: [w405] -> w392
                tunnel: [w404] -> w391
                tunnel: w388 -> [w403]
                tunnel: [w403] -> w385
                tunnel: w384 -> [w402]
                tunnel: [w402] -> w383
                tunnel: w380 -> [w401]
                tunnel: [w401] -> w378
                tunnel: w377 -> [w400]
                tunnel: [w400] -> w375
                tunnel: [w416] -> w390
                tunnel: w394 -> [w415]
                tunnel: w393 -> [w414]
                tunnel: w392 -> [w413]
                tunnel: w391 -> [w412]
                tunnel: [w411] -> w386
                tunnel: w385 -> [w411]
                tunnel: w383 -> [w410]
                tunnel: [w410] -> w382
                tunnel: [w409] -> w379
                tunnel: w378 -> [w409]
                tunnel: [w408] -> w376
                tunnel: w375 -> [w408]
                tunnel: w390 -> [w462]
                tunnel: [w462] -> w389
                tunnel: [w458] -> w387
                tunnel: w386 -> [w458]
                tunnel: w382 -> [w457]
                tunnel: [w457] -> w381
                tunnel: w379 -> [w456]
                tunnel: w376 -> [w455]
                tunnel: [w456] -> w374
                tunnel: [w455] -> w373
                tunnel: w389 -> [_]
                tunnel: w387 -> [w468]
                tunnel: w381 -> [w467]
                tunnel: w374 -> [w463]
                tunnel: w373 -> [w464]
                tunnel: [w466] -> w372
                tunnel: [w465] -> w371
                tunnel: [w464] -> w370
                tunnel: [w463] -> w369
                tunnel: [w586] -> w365
                tunnel: [w587] -> w366
                tunnel: [w588] -> w368
                tunnel: [w589] -> w367
                tunnel: w372 -> [w589]
                tunnel: w371 -> [w588]
                tunnel: w370 -> [w593]
                tunnel: w369 -> [w592]
                frame #0 {
                }
                frame #1 {
                  n168 = for {
                    tunnel: w413 -> [w426]
                    tunnel: w415 -> [w428]
                    tunnel: w412 -> [w425] mode=indexing
                    tunnel: [w427] -> w416
                    tunnel: w414 -> [w418]
                    i -> [w417]
                    n169 = call "Channel Status.vi"("All Channels (T)"=FALSE, "Channel"=w425, "BoardHandle"=w426) -> ("Channel Status Array"=w424:T3, "BoardHandle out"=w419:T5)  [unwired: 6 in, 1 out]
                    n170 = Index Array(array=w424, index=0) -> (element=w423:T6)
                    n171 = Unbundle By Name(w423) -> ("ON"=w421:bool)
                    n172 = case shown="True" w421 {
                      tunnel: w428 -> [w429 w436]
                      tunnel: [w429 w440] -> w427
                      tunnel: w419 -> [_ w435]
                      tunnel: w425 -> [_ w439]
                      tunnel: w418 -> [_ w438]
                      tunnel: w417 -> [_ w433]
                      frame False {
                      }
                      frame True {
                        n173 = Index Array(array="Vstop", index=w433) -> (element=w432:dbl)
                        n174 = call "Read out VSET.vi"("error in (no error)"=w436, "BoardHandle"=w435) -> ("Vset values (V)"=w434:dbl[])  [unwired: 6 in, 3 out]
                        n175 = Index Array(array=w434, index=w433) -> (element=w431:dbl)
                        n176 = Greater?(x=w432, y=w431) -> (0:w430:bool)
                        n177 = case shown="False" w430 {
                          tunnel: w436 -> [w441 w454]
                          tunnel: [w441 w453] -> w440
                          tunnel: w435 -> [_ w452]
                          tunnel: w439 -> [_ w451]
                          tunnel: w438 -> [_ w449]
                          tunnel: w433 -> [_ w444]
                          frame False {
                          }
                          frame True {
                            n178 = Index Array(array="Step [V]", index=w444) -> (element=w443:dbl)
                            n179 = Index Array(array="Vstart", index=w444) -> (element=w446:dbl)
                            n180 = Multiply(x=w443, y=w449) -> (x*y=w448:dbl)
                            n181 = Add(x=w446, y=w448) -> (x+y=w442:dbl)
                            n182 = call "Configure VSET.vi"("All Channels (F)"=FALSE, "error in (no error)"=w454, "Voltage Level (0.0 V)"=w442, "Channel (0)"=w451, "BoardHandle"=w452) -> ("error out"=w453:errorcluster)  [unwired: 5 in, 1 out]
                          }
                        }
                      }
                    }
                  }
                  n183 = local write "error out"(w416) -> ()
                }
                frame #2 {
                  n184 = Multiply(x="Waiting [s]", y=1000.0) -> (x*y=w459:dbl)
                  n185 = Wait (ms)(milliseconds to wait=w459) -> ()  [unwired: 1 out]
                }
                frame #3 {
                  n186 = for {
                    N: "pts/step" -> [_]
                    shift-right: [w473] -> w466
                    shift-left: w468 -> [w476]
                    shift-right: [w471] -> w465
                    shift-left: w467 -> [w475]
                    i -> [w479]
                    w477 = cluster{dbl[], dbl[]}[] []
                    w542 = FALSE ("Open/Close [T]")
                    n187 = Increment(x=w479) -> (x+1=→"logged pts/step":i32)
                    n188 = local read "Number of Channel Detected"() -> (w537:u8)
                    n189 = Get Date/Time In Seconds() -> (seconds since 1Jan1904=w540:timestamp)
                    n190 = local read "seconds since 1Jan1904"() -> (w470:timestamp)
                    n191 = local read "VISA resource name in"() -> (w545:refnum<visa-resource-name>)
                    n192 = local read "Module Address"() -> (w541:u16)
                    n193 = local read "VMON Array"() -> (w483:dbl[][])
                    n194 = local read "IMON Array"() -> (w482:dbl[][])
                    n195 = Subtract(x=w540, y=w470) -> (x-y=w538:dbl)
                    n196 = local read "Time Array"() -> (w539:dbl[])
                    n197 = Wait Until Next ms Multiple(millisecond multiple=u32 1000 ("milliseconds to wait")) -> ()  [unwired: 1 out]
                    n198 = Build Array (concatenate)(w539, w538) -> (w528:dbl[])
                    n199 = local write "Time Array"(w528) -> ()
                    n200 = local read "Save"() -> (w488:bool)
                    n201 = local read "error out"() -> (w517:errorcluster)
                    n202 = call "N1471A-MonitorVMON.vi"("VISA resource name in"=w545, "Module Address"=w541, "Channel"=w537, "error in (no error)"=w517, "Open/Close [T]"=w542) -> ("VISA resource name out"=w544:refnum<visa-resource-name>, "Values"=w480:string[], "error out"=w543:errorcluster)  [unwired: 9 in, 3 out]
                    n203 = call "N1471A-MonitorIMON.vi"("VISA resource name in"=w544, "Module Address"=w541, "Channel"=w537, "error in (no error)"=w543, "Open/Close [T]"=w542) -> ("Values"=w481:string[])  [unwired: 9 in, 5 out]
                    n204 = for {
                      N: w537 -> [_]
                      tunnel: w480 -> [w578] mode=indexing
                      tunnel: w481 -> [w577] mode=indexing
                      tunnel: [w572] -> w497 mode=indexing
                      tunnel: [w571] -> w508 mode=indexing
                      tunnel: w482 -> [w574]
                      tunnel: w483 -> [w576]
                      tunnel: w481 -> [_] mode=indexing
                      tunnel: w480 -> [_] mode=indexing
                      tunnel: [w567] -> w474 mode=indexing
                      tunnel: [w566] -> w472 mode=indexing
                      tunnel: w476 -> [w563]
                      tunnel: w475 -> [w562]
                      i -> [w565]
                      n205 = Index Array(array=w576, index (col)=w565) -> (element=w575:dbl[])  [unwired: 1 in]
                      n206 = Index Array(array=w574, index (col)=w565) -> (element=w573:dbl[])  [unwired: 1 in]
                      n207 = Index Array(array=w562, index (col)=w565) -> (element=w564:dbl[])  [unwired: 1 in]
                      n208 = Index Array(array=w563, index (col)=w565) -> (element=w570:dbl[])  [unwired: 1 in]
                      n209 = Fract/Exp String To Number(string=w578) -> (number=w569:dbl)  [unwired: 3 in, 1 out]
                      n210 = Fract/Exp String To Number(string=w577) -> (number=w568:dbl)  [unwired: 3 in, 1 out]
                      n211 = Build Array (concatenate)(w564, w568) -> (w566:dbl[])
                      n212 = Build Array (concatenate)(w570, w569) -> (w567:dbl[])
                      n213 = Build Array (concatenate)(w575, w569) -> (w572:dbl[])
                      n214 = Build Array (concatenate)(w573, w568) -> (w571:dbl[])
                    }
                    n215 = Multiply(x=w508, y=1000) -> (x*y=w507:dbl[][])
                    n216 = Index Array(array=w497, index (row) #1=0 ("index (row)"), index (row) #2=1 ("index (row)"), index (row) #3=2 ("index (row)"), index (row) #4=3 ("index (row)")) -> (element #1=w527:dbl[], element #2=w525:dbl[], element #3=w523:dbl[], element #4=w521:dbl[])  [unwired: 4 in]
                    n217 = Index Array(array=w508, index (row) #1=0 ("index (row)"), index (row) #2=1 ("index (row)"), index (row) #3=2 ("index (row)"), index (row) #4=3 ("index (row)")) -> (element #1=w526:dbl[], element #2=w524:dbl[], element #3=w522:dbl[], element #4=w520:dbl[])  [unwired: 4 in]
                    n218 = Transpose 2D Array(2D array=w497) -> (transposed array=w485:dbl[][])
                    n219 = Transpose 2D Array(2D array=w508) -> (transposed array=w484:dbl[][])
                    n220 = Transpose 2D Array(2D array=w474) -> (transposed array=w473:dbl[][])
                    n221 = Transpose 2D Array(2D array=w472) -> (transposed array=w471:dbl[][])
                    n222 = Index Array(array=w507, index (row) #1=0 ("index (row)"), index (row) #2=1 ("index (row)"), index (row) #3=2 ("index (row)"), index (row) #4=3 ("index (row)")) -> (element #1=w512:dbl[], element #2=w511:dbl[], element #3=w510:dbl[], element #4=w509:dbl[])  [unwired: 4 in]
                    n223 = Build Array(w528, w527, w526, w525, w524, w523, w522, w521, w520) -> (w519:dbl[][])
                    n224 = local write "VMON Array"(w485) -> ()
                    n225 = local write "IMON Array"(w484) -> ()
                    n226 = Reverse 1D Array(array=w512) -> (reversed array=w492:dbl[])
                    n227 = Reverse 1D Array(array=w511) -> (reversed array=w491:dbl[])
                    n228 = Reverse 1D Array(array=w510) -> (reversed array=w490:dbl[])
                    n229 = Reverse 1D Array(array=w509) -> (reversed array=w489:dbl[])
                    n230 = local write "IMON RT 2"(w491) -> ()
                    n231 = case shown="False" w488 {
                      tunnel: w519 -> [_ w546]
                      frame False {
                      }
                      frame True {
                        n232 = flat-sequence {
                          tunnel: w546 -> [w548]
                          frame #0 {
                            n233 = call-poly <vilib>:"Write To Spreadsheet File.vi"("transpose? (no:F)"=TRUE, "format (%.3f)"="%.5f", "2D data"=w548) -> ()  [unwired: 5 in, 1 out]
                          }
                          frame #1 {
                            n234 = local write "Save"(FALSE ("Save")) -> ()
                          }
                        }
                      }
                    }
                    n235 = local write "IMON RT 1"(w492) -> ()
                    n236 = local write "IMON RT 4"(w489) -> ()
                    n237 = local write "IMON RT 3"(w490) -> ()
                    n238 = for {
                      tunnel: w497 -> [w552] mode=indexing
                      shift-right: [w561] -> w487
                      shift-left: w477 -> [w560]
                      shift-right: [w559] -> w486
                      shift-left: w477 -> [w558]
                      tunnel: w508 -> [w557] mode=indexing
                      tunnel: w528 -> [w553]
                      n239 = Multiply(x=w557, y=1000) -> (x*y=w551:dbl[])
                      n240 = Bundle(w553, w552) -> (w556:cluster{dbl[], dbl[]})  [unwired: 1 in]
                      n241 = Bundle(w553, w551) -> (w555:cluster{dbl[], dbl[]})  [unwired: 1 in]
                      n242 = Build Array (concatenate)(w560, w556) -> (w561:cluster{dbl[], dbl[]}[])
                      n243 = Build Array (concatenate)(w558, w555) -> (w559:cluster{dbl[], dbl[]}[])
                    }
                    n244 = Index Array(array=w497, index (row) #1=0 ("index (row)"), index (row) #2=1 ("index (row)"), index (row) #3=2 ("index (row)"), index (row) #4=3 ("index (row)")) -> (element #1=w501:dbl[], element #2=w500:dbl[], element #3=w499:dbl[], element #4=w498:dbl[])  [unwired: 4 in]
                    n245 = local write "VMon Graph"(w487) -> ()
                    n246 = Reverse 1D Array(array=w501) -> (reversed array=w496:dbl[])
                    n247 = Reverse 1D Array(array=w500) -> (reversed array=w495:dbl[])
                    n248 = Reverse 1D Array(array=w499) -> (reversed array=w494:dbl[])
                    n249 = Reverse 1D Array(array=w498) -> (reversed array=w493:dbl[])
                    n250 = local write "IMon Graph"(w486) -> ()
                    n251 = local write "VMON RT 4"(w493) -> ()
                    n252 = local write "VMON RT 2"(w495) -> ()
                    n253 = local write "VMON RT 1"(w496) -> ()
                    n254 = local write "VMON RT 3"(w494) -> ()
                  }
                }
                frame #4 {
                  n255 = for {
                    tunnel: w589 -> [w629]
                    tunnel: w588 -> [w624]
                    tunnel: w592 -> [w617] mode=indexing
                    tunnel: [w628] -> w587 mode=indexing
                    tunnel: w593 -> [w616] mode=indexing
                    tunnel: [w621] -> w586 mode=indexing
                    i -> [w623]
                    w620 = 0 items=["standard deviation", "range", "mean absolute deviation", "interquartile range"] ("type")
                    n256 = Index Array(array=w629, index (col)=w623) -> (element=w618:dbl[])  [unwired: 1 in]
                    n257 = Index Array(array=w624, index (col)=w623) -> (element=w619:dbl[])  [unwired: 1 in]
                    n258 = local read "logged pts/step"() -> (w626:i32)
                    n259 = Reverse 1D Array(array=w618) -> (reversed array=w632:dbl[])
                    n260 = Reverse 1D Array(array=w619) -> (reversed array=w627:dbl[])
                    n261 = Array Subset(array=w627, length=w626) -> (w625:dbl[])  [unwired: 1 in]
                    n262 = Array Subset(array=w632, length=w626) -> (w631:dbl[])  [unwired: 1 in]
                    n263 = call-poly <vilib>:"Mean.vi"("X"=w631) -> ("mean"=w630:dbl)  [unwired: 1 out]
                    n264 = call <vilib>:"Measures of Spread.vi"("x array"=w631) -> ()  [unwired: 9 in, 2 out]
                    n265 = call-poly <vilib>:"Mean.vi"("X"=w625) -> ("mean"=w622:dbl)  [unwired: 1 out]
                    n266 = call <vilib>:"Measures of Spread.vi"("type"=w620, "x array"=w625) -> ()  [unwired: 8 in, 2 out]
                    n267 = Build Array (concatenate)(w616, w622) -> (w621:dbl[])
                    n268 = Build Array (concatenate)(w617, w630) -> (w628:dbl[])
                  }
                  n269 = Transpose 2D Array(2D array=w589) -> (transposed array=w581:dbl[][])
                  n270 = Transpose 2D Array(2D array=w588) -> (transposed array=w579:dbl[][])
                  n271 = for {
                    N: 3 -> [_]
                    tunnel: w581 -> [w598] mode=indexing
                    tunnel: [w598] -> w582
                  }
                  n272 = for {
                    N: 2 -> [_]
                    tunnel: w581 -> [w599] mode=indexing
                    tunnel: [w599] -> w583
                  }
                  n273 = Subtract(x=w583, y=w582) -> (x-y=w580:dbl[])
                  n274 = for {
                    tunnel: w580 -> [w615]
                    tunnel: w579 -> [w610] mode=indexing
                    shift-right: [w612] -> w591
                    shift-left: cluster{dbl[], dbl[]}[] [] ("plot data") -> [w613]
                    n275 = Multiply(x=w610, y=1000) -> (x*y=w609:dbl[])
                    n276 = Bundle(w615, w609) -> (w614:cluster{dbl[], dbl[]})  [unwired: 1 in]
                    n277 = Build Array (concatenate)(w613, w614) -> (w612:cluster{dbl[], dbl[]}[])
                  }
                  n278 = for {
                    tunnel: w587 -> [w606] mode=indexing
                    tunnel: w586 -> [w601] mode=indexing
                    shift-right: [w603] -> w597
                    shift-left: cluster{dbl[], dbl[]}[] [] -> [w604]
                    n279 = Multiply(x=w601, y=1000) -> (x*y=w600:dbl[])
                    n280 = Bundle(w606, w600) -> (w605:cluster{dbl[], dbl[]})  [unwired: 1 in]
                    n281 = Build Array (concatenate)(w604, w605) -> (w603:cluster{dbl[], dbl[]}[])
                  }
                  n282 = local read "Average values"() -> (w595:bool)
                  n283 = case shown="False" w595 {
                    tunnel: w591 -> [w607 _]
                    tunnel: [w607 w608] -> w596
                    tunnel: w597 -> [_ w608]
                    frame False {
                    }
                    frame True {
                    }
                  }
                  "Scatter Plot" <- w596
                }
              }
            }
          }
          event "Update On/OFF": Mouse Down {
            n284 = event-data() -> ()  [unwired: 1 in, 7 out]
            n285 = local read "Number of Channel Detected"() -> (w641:u8)
            n286 = local read "Channels Selection"() -> (w646:bool[])
            n287 = local read "VISA resource name in"() -> (w648:refnum<visa-resource-name>)
            n288 = local read "Module Address"() -> (w647:u16)
            n289 = local read "error out"() -> (w649:errorcluster)
            n290 = Array Subset(array=u8[] [0, 1, 2, 3], index=0, length=w641) -> (w654:u8[])
            n291 = And Array Elements(Boolean array=w646) -> (logical AND=w652:bool)
            n292 = for {
              shift-right: [w802] -> w651
              shift-left: u8[] [] -> [w803]
              tunnel: w654 -> [w801] mode=indexing
              tunnel: w646 -> [w800] mode=indexing
              shift-right: [w798] -> w642
              shift-left: bool[] [] -> [w797]
              tunnel: "Channels ON/OFF" -> [w799] mode=indexing
              n293 = case shown="True" w800 {
                tunnel: w803 -> [w805 w811]
                tunnel: [w805 w810] -> w802
                tunnel: w801 -> [_ w809]
                tunnel: w799 -> [_ w808]
                tunnel: [w804 w807] -> w798
                tunnel: w797 -> [w804 w806]
                frame False {
                }
                frame True {
                  n294 = Build Array (concatenate)(w806, w808) -> (w807:bool[])
                  n295 = Build Array (concatenate)(w811, w809) -> (w810:u8[])
                }
              }
            }
            n296 = case shown="True" w652 {
              tunnel: w641 -> [_ w695]
              tunnel: w651 -> [w664 w687]
              tunnel: [w663 w699] -> w650
              tunnel: w649 -> [w662 w698]
              tunnel: w648 -> [w661 w697]
              tunnel: w647 -> [w660 w696]
              tunnel: w642 -> [w659 _]
              tunnel: "Channels ON/OFF" -> [_ w691]
              tunnel: [w657 w689] -> w643
              tunnel: w642 -> [_ w686]
              frame False {
                n297 = for {
                  tunnel: w664 -> [w670] mode=indexing
                  shift-right: [w666] -> w663
                  shift-left: w662 -> [w667]
                  tunnel: w661 -> [w668]
                  tunnel: w660 -> [w669]
                  tunnel: w659 -> [w671] mode=indexing
                  tunnel: [w665] -> w658 mode=indexing
                  n298 = case shown="False" w671 {
                    tunnel: w670 -> [w675 w685]
                    tunnel: w669 -> [w676 w684]
                    tunnel: w668 -> [w677 w683]
                    tunnel: w667 -> [w674 w682]
                    tunnel: [w673 w681] -> w666
                    tunnel: [w672 w679] -> w665
                    frame False {
                      n299 = call "N1471A-SetChOFF.vi"("VISA resource name in"=w677, "Module Address"=w676, "Channel"=w675, "error in (no error)"=w674, "Open/Close [T]"=FALSE) -> ("Error"=w672:bool, "error out"=w673:errorcluster)  [unwired: 9 in, 4 out]
                    }
                    frame True {
                      n300 = call "N1471A-SetChON.vi"("VISA resource name in"=w683, "Module Address"=w684, "Channel"=w685, "error in (no error)"=w682, "Open/Close [T]"=FALSE) -> ("Error"=w679:bool, "error out"=w681:errorcluster)  [unwired: 9 in, 4 out]
                    }
                  }
                }
                n301 = Or Array Elements(Boolean array=w658) -> (logical OR=w657:bool)
              }
              frame True {
                n302 = Boolean To (0,1)(Boolean=w691) -> (0, 1=w694:i16[])
                n303 = And Array Elements(Boolean array=w691) -> (logical AND=w690:bool)
                n304 = Array Max & Min(array=w694) -> (max value=w693:i16, min value=w688:i16)  [unwired: 2 out]
                n305 = Equal?(x=w693, y=w688) -> (x = y?=w692:bool)
                n306 = case shown="False" w692 {
                  tunnel: [w710 w782] -> w699
                  tunnel: w698 -> [w712 w781]
                  tunnel: w697 -> [w709 w780]
                  tunnel: w696 -> [w706 w779]
                  tunnel: w695 -> [w705 w778]
                  tunnel: w690 -> [_ w777]
                  tunnel: [w704 w776] -> w689
                  tunnel: w687 -> [w702 _]
                  tunnel: w686 -> [w701 _]
                  frame False {
                    n307 = call "Prompt User for Input"("error in (no error)"=w712) -> ("DO IT ANYWAY"=w700:bool, "OFF"=w707:bool, "ON"=w708:bool, "OK"=w703:bool, "error out"=w711:errorcluster)  [unwired: 14 in]
                    n308 = case shown="False" w700 {
                      tunnel: w711 -> [w723 w750]
                      tunnel: [w722 w749] -> w710
                      tunnel: w709 -> [w721 w752]
                      tunnel: w708 -> [w720 _]
                      tunnel: w707 -> [w719 _]
                      tunnel: w706 -> [w716 w751]
                      tunnel: w705 -> [w715 _]
                      tunnel: [w714 w747] -> w704
                      tunnel: w703 -> [w713 _]
                      tunnel: w702 -> [_ w754]
                      tunnel: w701 -> [_ w753]
                      frame False {
                        n309 = Not(x=w719) -> (.not. x?=w718:bool)
                        n310 = Compound Arithmetic op=AND(w720, w718) -> (w717:bool)
                        n311 = case shown="True" w713 {
                          tunnel: w723 -> [w725 w732]
                          tunnel: [w725 w731] -> w722
                          tunnel: w721 -> [_ w730]
                          tunnel: w717 -> [_ w729]
                          tunnel: w716 -> [_ w728]
                          tunnel: w715 -> [_ w727]
                          tunnel: [FALSE ("Open/Close [T]") w726] -> w714
                          frame False {
                          }
                          frame True {
                            n312 = case shown="False" w729 {
                              tunnel: w727 -> [w735 w746]
                              tunnel: w728 -> [w736 w745]
                              tunnel: w730 -> [w737 w744]
                              tunnel: w732 -> [w739 w743]
                              tunnel: [w738 w742] -> w731
                              tunnel: [w733 w740] -> w726
                              frame False {
                                n313 = call "N1471A-SetChOFF.vi"("VISA resource name in"=w737, "Module Address"=w736, "Channel"=w735, "error in (no error)"=w739, "Open/Close [T]"=FALSE) -> ("Error"=w733:bool, "error out"=w738:errorcluster)  [unwired: 9 in, 4 out]
                              }
                              frame True {
                                n314 = call "N1471A-SetChON.vi"("VISA resource name in"=w744, "Module Address"=w745, "Channel"=w746, "error in (no error)"=w743, "Open/Close [T]"=FALSE) -> ("Error"=w740:bool, "error out"=w742:errorcluster)  [unwired: 9 in, 4 out]
                              }
                            }
                          }
                        }
                      }
                      frame True {
                        n315 = for {
                          tunnel: w754 -> [w758] mode=indexing
                          tunnel: w753 -> [w761] mode=indexing
                          tunnel: w752 -> [w760]
                          tunnel: w751 -> [w759]
                          tunnel: [w755] -> w748 mode=indexing
                          shift-right: [w756] -> w749
                          shift-left: w750 -> [w757]
                          n316 = case shown="False" w761 {
                            tunnel: w760 -> [w767 w775]
                            tunnel: w759 -> [w766 w774]
                            tunnel: w758 -> [w765 w773]
                            tunnel: w757 -> [w764 w772]
                            tunnel: [w763 w771] -> w756
                            tunnel: [w762 w770] -> w755
                            frame False {
                              n317 = call "N1471A-SetChOFF.vi"("VISA resource name in"=w767, "Module Address"=w766, "Channel"=w765, "error in (no error)"=w764, "Open/Close [T]"=FALSE) -> ("Error"=w762:bool, "error out"=w763:errorcluster)  [unwired: 9 in, 4 out]
                            }
                            frame True {
                              n318 = call "N1471A-SetChON.vi"("VISA resource name in"=w775, "Module Address"=w774, "Channel"=w773, "error in (no error)"=w772, "Open/Close [T]"=FALSE) -> ("Error"=w770:bool, "error out"=w771:errorcluster)  [unwired: 9 in, 4 out]
                            }
                          }
                        }
                        n319 = Or Array Elements(Boolean array=w748) -> (logical OR=w747:bool)
                      }
                    }
                  }
                  frame True {
                    n320 = case shown="False" w777 {
                      tunnel: w778 -> [w785 w796]
                      tunnel: w779 -> [w786 w795]
                      tunnel: w780 -> [w787 w794]
                      tunnel: w781 -> [w789 w793]
                      tunnel: [w788 w792] -> w782
                      tunnel: [w783 w790] -> w776
                      frame False {
                        n321 = call "N1471A-SetChOFF.vi"("VISA resource name in"=w787, "Module Address"=w786, "Channel"=w785, "error in (no error)"=w789, "Open/Close [T]"=FALSE) -> ("Error"=w783:bool, "error out"=w788:errorcluster)  [unwired: 9 in, 4 out]
                      }
                      frame True {
                        n322 = call "N1471A-SetChON.vi"("VISA resource name in"=w794, "Module Address"=w795, "Channel"=w796, "error in (no error)"=w793, "Open/Close [T]"=FALSE) -> ("Error"=w790:bool, "error out"=w792:errorcluster)  [unwired: 9 in, 4 out]
                      }
                    }
                  }
                }
              }
            }
            "Error  on \nChannels \nON/OFF" <- w643
            n323 = local write "error out"(w650) -> ()
          }
          event "ALL ON": Mouse Down {
            w815 = TRUE ("All Channels (F)")
            n324 = event-data() -> ()  [unwired: 1 in, 7 out]
            n325 = local read "Board Handle"() -> (w814:T1)
            n326 = local read "error out"() -> (w813:errorcluster)
            n327 = call "Channel Power Enable.vi"("All Channels (F)"=w815, "error in (no error)"=w813, "Enable (OFF)"=w815, "BoardHandle"=w814) -> ("error out"=w812:errorcluster)  [unwired: 6 in, 1 out]
            n328 = local write "error out"(w812) -> ()
          }
          event "ALL OFF": Mouse Down {
            n329 = event-data() -> ()  [unwired: 1 in, 7 out]
            n330 = local read "Board Handle"() -> (w820:T1)
            n331 = local read "error out"() -> (w819:errorcluster)
            n332 = call "Channel Power Enable.vi"("All Channels (F)"=TRUE, "error in (no error)"=w819, "Enable (OFF)"=FALSE ("Open/Close [T]"), "BoardHandle"=w820) -> ("error out"=w816:errorcluster)  [unwired: 6 in, 1 out]
            n333 = local write "error out"(w816) -> ()
          }
        }
      }
      frame Error {
      }
    }
    n334 = local write "error out"(w23) -> ()
    n335 = call <vilib>:"Simple Error Handler.vi"("error in (no error)"=w23) -> ("error?"=w27:bool)  [unwired: 4 in, 4 out]
    n336 = Compound Arithmetic op=OR(w27, "stop") -> (w26:bool)
  }
  n337 = local read "VISA resource name in"() -> (w3:refnum<visa-resource-name>)
  n338 = local write "stop"(w15) -> ()
  n339 = call "Close.vi"("error in (no error)"=w4, "VISA resource name"=w3) -> ("error out"=→"error out":errorcluster)  [unwired: 9 in]
  "seconds since 1Jan1904" <- w1
